vi "CMC_Homework_09.vi"(11 "FILE FORMAT":enum16{"ASCII", "BIN", "TDMS"}(ring)) -> (0 "Error Out":errorcluster, 1 "Time TMDS (s)":dbl, 2 "Time Binary (s)":dbl, 3 "Time ASCII (s)":dbl)   [LabVIEW 2013]
panel:
  # "ASCII representation is larger than the data itself for non-text and causes the program to run slower add to that position keeping.\nBinary files store numerics easily because any number from 0 to 4 billion still takes up four bytes for each number no matter the size.\nTDMS files use binary to store and then xml to configure the position and require two different files. This means for lots of lines of data\nit takes more time to write all the positions down."
  # "10,000 x 1000 Matrix File Write Times:\nASCII   29.111\nBIN      2.149\nTDMS  1.52"
  # "100,000 x 1 Matrix File Write Times:\nASCII   5.365\nBIN      4.244\nTDMS  9.214"
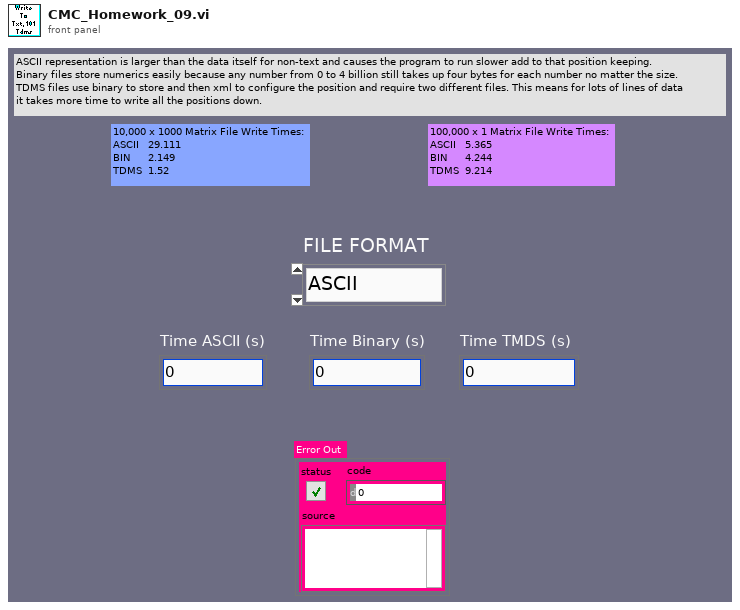
[diagram p1: front panel]
types:
  T1 = enum16{"open", "replace", "create", "open or create", "replace or create", "replace or create with confirmation"}
  T2 = enum16{"open", "open or create", "create or replace", "create", "open (read-only)"}
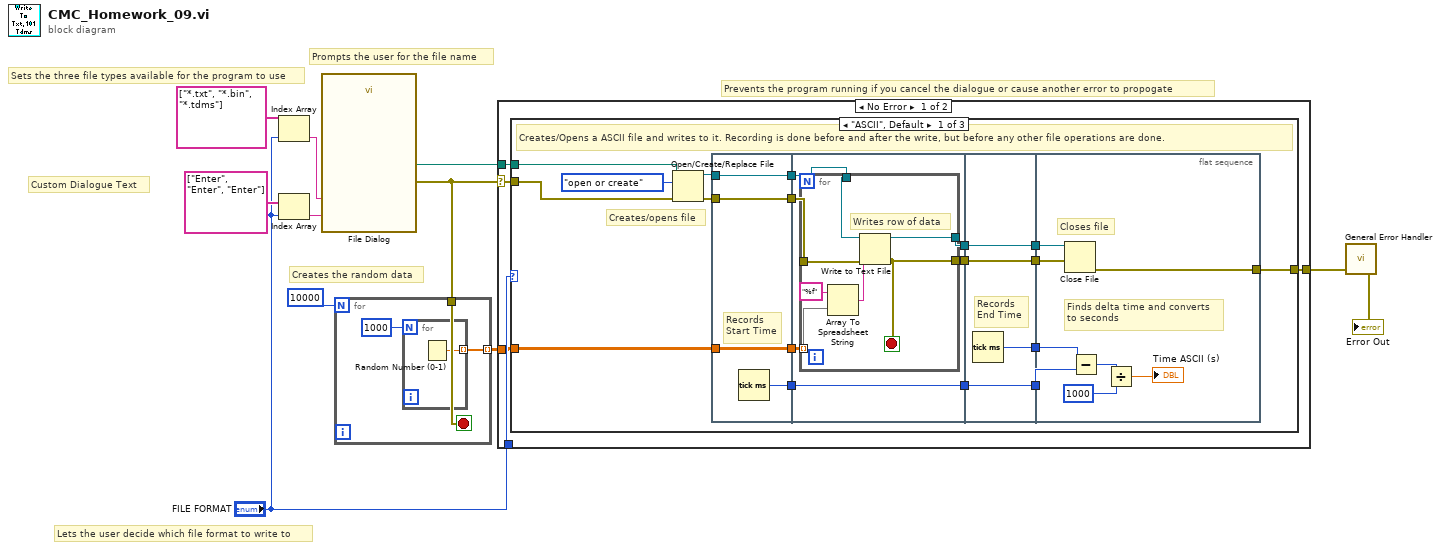
[diagram p0: block diagram]
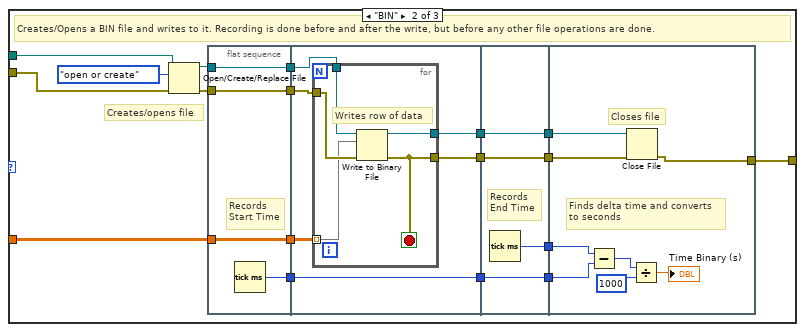
[diagram p2: hidden frame]
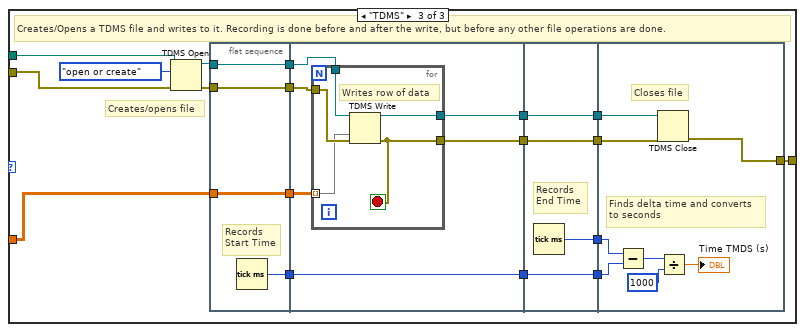
[diagram p3: hidden frame]
diagram:
  # "Custom Dialogue Text"
  # "Creates the random data"
  # "Lets the user decide which file format to write to"
  # "Sets the three file types available for the program to use"
  # "Prompts the user for the file name"
  # "Prevents the program running if you cancel the dialogue or cause another error to propogate"
  n1 = Index Array(array=string[] ["*.txt", "*.bin", "*.tdms"], index="FILE FORMAT") -> (element=w8:string)
  n2 = Index Array(array=string[] ["Enter", "Enter", "Enter"], index="FILE FORMAT") -> (element=w7:string)
  n3 = call "File Dialog"("prompt"=w7, "pattern (all files)"=w8) -> ("selected path"=w5:path, "error out"=w2:errorcluster)  [unwired: 10 in, 2 out]
  n4 = for {
    N: 10000 -> [_]
    tunnel: [w12] -> w1 mode=indexing
    tunnel: w2 -> [w11]
    stop <- w11 stop-if-true
    n5 = for {
      N: 1000 -> [_]
      tunnel: [w14] -> w12 mode=indexing
      n6 = Random Number (0-1)() -> (number: 0 to 1=w14:dbl)
    }
  }
  n7 = case shown="No Error" w2 {
    selector: w2 -> [w18 w157]
    tunnel: w5 -> [w19 _]
    tunnel: [w15 w157] -> w4
    tunnel: "FILE FORMAT" -> [w17 _]
    tunnel: w1 -> [w16 _]
    frame No Error {
      n8 = case shown="\"ASCII\", Default" w17 {
        tunnel: w19 -> [w30 w81 w123]
        tunnel: w18 -> [w29 w79 w122]
        tunnel: w16 -> [w27 w75 w118]
        tunnel: [w21 w68 w112] -> w15
        frame "ASCII", Default {
          # "Creates/opens file"
          # "Creates/Opens a ASCII file and writes to it. Recording is done before and after the write, but before any other file operations are done."
          n9 = Open/Create/Replace File(file path (use dialog)=w30, error in=w29, operation (0:open)=T1."open or create") -> (refnum out=w31:refnum<file>, error out=w32:errorcluster)  [unwired: 3 in, 1 out]
          n10 = flat-sequence {
            tunnel: [w41] -> w37
            tunnel: w32 -> [w39]
            tunnel: [w40] -> w36
            tunnel: w31 -> [w40]
            tunnel: [w39] -> w35
            tunnel: [w38] -> w28
            tunnel: w27 -> [w38]
            tunnel: [w47] -> w34
            tunnel: w37 -> [w47]
            tunnel: w36 -> [w45]
            tunnel: w35 -> [w44]
            tunnel: w28 -> [w46]
            tunnel: [w43] -> w25
            tunnel: [w42] -> w22
            tunnel: w34 -> [w55]
            tunnel: [w58] -> w26
            tunnel: w25 -> [w57]
            tunnel: [w57] -> w24
            tunnel: [w56] -> w23
            tunnel: w22 -> [w56]
            tunnel: [w55] -> w20
            tunnel: w26 -> [w63]
            tunnel: w24 -> [w66]
            tunnel: w23 -> [w65]
            tunnel: [w64] -> w21
            tunnel: w20 -> [w62]
            frame #0 {
              # "Records\nStart Time"
              n11 = Tick Count (ms)() -> (millisecond timer value=w41:u32)
            }
            frame #1 {
              n12 = for {
                tunnel: w46 -> [w54] mode=indexing
                tunnel: w45 -> [w51]
                tunnel: w44 -> [w53]
                tunnel: [w50] -> w42
                tunnel: [w49] -> w43
                stop <- w50 stop-if-true
                # "Writes row of data"
                n13 = Array To Spreadsheet String(array=w54, 3:"%f" ("format string")) -> (spreadsheet string=w52:string)  [unwired: 1 in]
                n14 = Write to Text File(file (use dialog)=w51, text=w52, error in=w53) -> (refnum out=w49:refnum<file>, error out=w50:errorcluster)  [unwired: 1 in, 1 out]
              }
            }
            frame #2 {
              # "Records\nEnd Time"
              n15 = Tick Count (ms)() -> (millisecond timer value=w58:u32)
            }
            frame #3 {
              # "Closes file"
              # "Finds delta time and converts\nto seconds"
              n16 = Close File(refnum=w66, error in=w65) -> (error out=w64:errorcluster)  [unwired: 1 out]
              n17 = Subtract(x=w63, y=w62) -> (x-y=w60:u32)
              n18 = Divide(x=w60, y=u16 1000) -> (x/y=→"Time ASCII (s)":dbl)
            }
          }
        }
        frame "BIN" {
          # "Creates/opens file"
          # "Creates/Opens a BIN file and writes to it. Recording is done before and after the write, but before any other file operations are done."
          n19 = Open/Create/Replace File(file path (use dialog)=w81, error in=w79, operation (0:open)=T1."open or create") -> (refnum out=w77:refnum<file>, error out=w78:errorcluster)  [unwired: 3 in, 1 out]
          n20 = flat-sequence {
            tunnel: [w88] -> w84
            tunnel: w78 -> [w86]
            tunnel: [w87] -> w83
            tunnel: w77 -> [w87]
            tunnel: [w86] -> w76
            tunnel: w75 -> [w85]
            tunnel: [w85] -> w72
            tunnel: [w94] -> w82
            tunnel: w84 -> [w94]
            tunnel: w83 -> [w93]
            tunnel: w76 -> [w92]
            tunnel: [w91] -> w74
            tunnel: [w90] -> w73
            tunnel: w72 -> [w89]
            tunnel: w82 -> [w100]
            tunnel: w74 -> [w102]
            tunnel: w73 -> [w101]
            tunnel: [w103] -> w71
            tunnel: [w102] -> w70
            tunnel: [w101] -> w69
            tunnel: [w100] -> w67
            tunnel: w71 -> [w108]
            tunnel: w70 -> [w111]
            tunnel: w69 -> [w110]
            tunnel: [w109] -> w68
            tunnel: w67 -> [w107]
            frame #0 {
              # "Records\nStart Time"
              n21 = Tick Count (ms)() -> (millisecond timer value=w88:u32)
            }
            frame #1 {
              n22 = for {
                tunnel: w93 -> [w97]
                tunnel: w92 -> [w99]
                tunnel: [w98] -> w90
                tunnel: [w96] -> w91
                tunnel: w89 -> [w95] mode=indexing
                stop <- w98 stop-if-true
                # "Writes row of data"
                n23 = Write to Binary File(file (use dialog)=w97, data=w95, error in=w99) -> (refnum out=w96:refnum<file>, error out=w98:errorcluster)  [unwired: 3 in, 1 out]
              }
            }
            frame #2 {
              # "Records\nEnd Time"
              n24 = Tick Count (ms)() -> (millisecond timer value=w103:u32)
            }
            frame #3 {
              # "Finds delta time and converts\nto seconds"
              # "Closes file"
              n25 = Subtract(x=w108, y=w107) -> (x-y=w105:u32)
              n26 = Close File(refnum=w111, error in=w110) -> (error out=w109:errorcluster)  [unwired: 1 out]
              n27 = Divide(x=w105, y=u32 1000) -> (x/y=→"Time Binary (s)":dbl)
            }
          }
        }
        frame "TDMS" {
          # "Creates/opens file"
          # "Creates/Opens a TDMS file and writes to it. Recording is done before and after the write, but before any other file operations are done."
          n28 = TDMS Open(8:w122, 10:T2."open or create" ("operation (0:open)"), 11:w123) -> (0:w125:errorcluster, 3:w124:refnum<k34>)  [unwired: 4 in]
          n29 = flat-sequence {
            tunnel: [w133] -> w129
            tunnel: w125 -> [w131]
            tunnel: [w132] -> w128
            tunnel: w124 -> [w132]
            tunnel: [w131] -> w127
            tunnel: [w130] -> w119
            tunnel: w118 -> [w130]
            tunnel: [w139] -> w126
            tunnel: w129 -> [w139]
            tunnel: w128 -> [w138]
            tunnel: w127 -> [w137]
            tunnel: [w136] -> w120
            tunnel: w119 -> [w135]
            tunnel: [w134] -> w114
            tunnel: w126 -> [w147]
            tunnel: w120 -> [w145]
            tunnel: [w148] -> w117
            tunnel: [w147] -> w116
            tunnel: [w146] -> w115
            tunnel: w114 -> [w146]
            tunnel: [w145] -> w113
            tunnel: w117 -> [w155]
            tunnel: w116 -> [w156]
            tunnel: w115 -> [w151]
            tunnel: w113 -> [w150]
            tunnel: [w149] -> w112
            frame #0 {
              # "Records\nStart Time"
              n30 = Tick Count (ms)() -> (millisecond timer value=w133:u32)
            }
            frame #1 {
              n31 = for {
                tunnel: w138 -> [w143]
                tunnel: w137 -> [w144]
                tunnel: [w142] -> w136
                tunnel: w135 -> [w141] mode=indexing
                tunnel: [w140] -> w134
                stop <- w142 stop-if-true
                # "Writes row of data"
                n32 = TDMS Write(0:w143, 9:w141, 11:w144) -> (4:w140:refnum<k34>, 15:w142:errorcluster)  [unwired: 3 in, 2 out]
              }
            }
            frame #2 {
              # "Records\nEnd Time"
              n33 = Tick Count (ms)() -> (millisecond timer value=w148:u32)
            }
            frame #3 {
              # "Closes file"
              # "Finds delta time and converts\nto seconds"
              n34 = Subtract(x=w155, y=w156) -> (x-y=w154:u32)
              n35 = TDMS Close(8:w150, 11:w151) -> (0:w149:errorcluster)  [unwired: 1 out]
              n36 = Divide(x=w154, y=1000) -> (x/y=→"Time TMDS (s)":dbl)
            }
          }
        }
      }
    }
    frame Error {
      # "Wires previous error all the way through"
    }
  }
  "Error Out" <- w4
  n37 = call <vilib>:"General Error Handler.vi"("error in (no error)"=w4) -> ()  [unwired: 10 in, 5 out]
